vi "Template Build All.vi"(9 "Build Options":T1, 10 "Changes":string, 11 "Version Increment":T3) -> (1 "Build Error":bool, 2 "Status":string, 3 "Version":T2, 5 "Description":string)   [LabVIEW 2021]
uses:
  <vilib>/CIF Foundation/CIF LabVIEW Scripting/LV Scripting/Typedef/Version Increment.ctl
  <vilib>/CIF Foundation/CIF LabVIEW Scripting/LV Scripting/Typedef/Version.ctl
  Template Core Utilities/Typedef/Build Options.ctl
  Template Core Utilities/TemplateCoreUtilities.lvlib
  <vilib>/CIF Foundation/CIF LabVIEW Scripting/LV Scripting/LV Scripting Utilities.lvlib
panel:
  # "If built RT plugin has problems loading you may need to change the settings in the build spec for the RT plugin. These settings optimize memory footprint but can cause load issues in some cases."
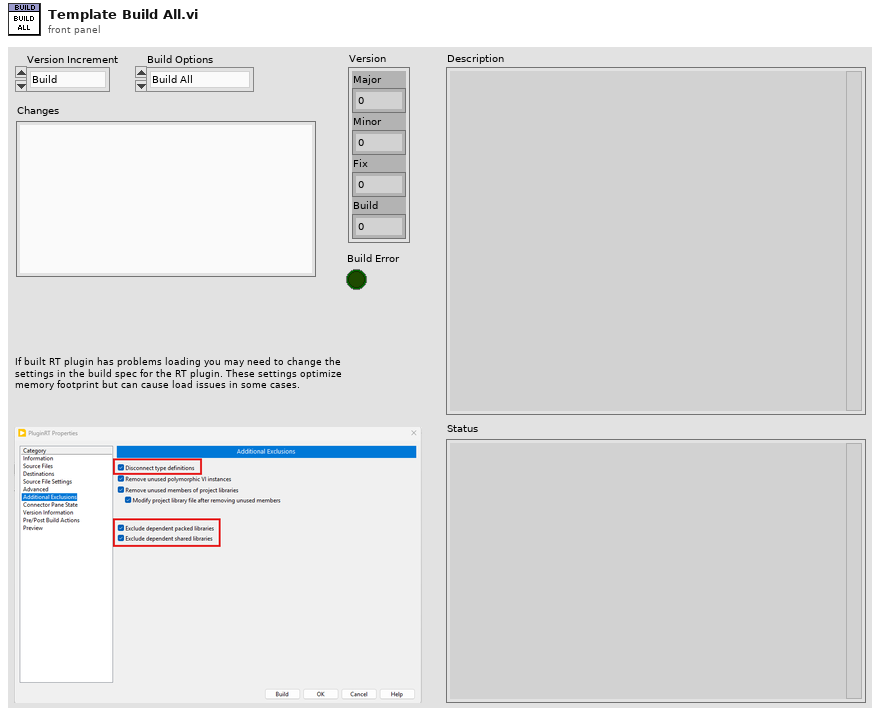
[diagram p1: front panel]
types:
  T1 = typedef "TemplateCoreUtilities.lvlib/Build Options.ctl" = enum16{"Build All", "Build RT Only", "Build Win Only", "Build UI Only"}
  T2 = typedef "Version.ctl" = cluster{"Major":u16, "Minor":u16, "Fix":u16, "Build":u16}
  T3 = typedef "LV Scripting Utilities.lvlib/Version Increment.ctl" = enum16{"Build", "Fix", "Minor", "Major"}
  T4 = typedef "TemplateCoreUtilities.lvlib/Calling VI References.ctl" = cluster{"Status":refnum<vi>, "Calling VI":refnum<vi>, "Description":refnum<vi>, "Version":refnum<vi>}
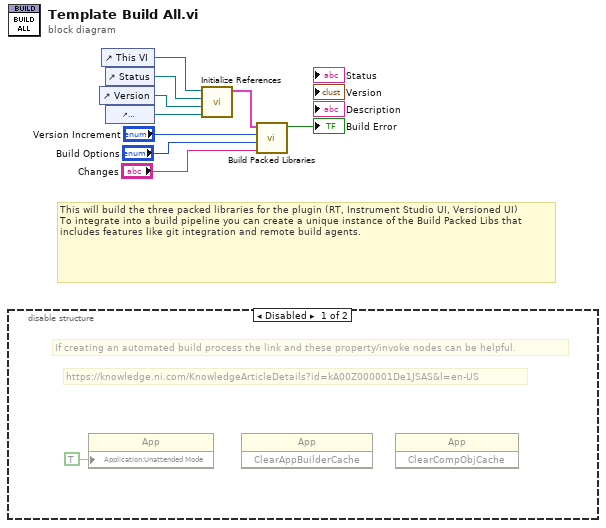
[diagram p0: block diagram]
diagram:
  # "This will build the three packed libraries for the plugin (RT, Instrument Studio UI, Versioned UI)\nTo integrate into a build pipeline you can create a unique instance of the Build Packed Libs that includes features like git integration and remote build agents."
  n1 = disable-structure shown="Disabled" {
    frame Disabled {
      # "If creating an automated build process the link and these property/invoke nodes can be helpful."
      # "https://knowledge.ni.com/KnowledgeArticleDetails?id=kA00Z000001De1JSAS&l=en-US"
      n2 = property class="App"("Application:Unattended Mode"=TRUE) -> ()  [unwired: 2 in, 2 out]
      n3 = invoke class="App" method="ClearAppBuilderCache"() -> ()  [unwired: 3 in, 3 out]
      n4 = invoke class="App" method="ClearCompObjCache"() -> ()  [unwired: 3 in, 3 out]
    }
    frame Enabled {
    }
  }
  n5 = control-ref of="Version"() -> (w7:refnum<vi>)
  n6 = control-ref of="This VI"() -> (w9:refnum<vi>)
  n7 = control-ref of="Status"() -> (w8:refnum<vi>)
  n8 = control-ref of="Description"() -> (w6:refnum<vi>)
  n9 = call "Initialize References.vi"("Description"=w6, "Version"=w7, "Status"=w8, "Calling VI"=w9) -> ("Calling VI References"=w5:T4)  [unwired: 7 in]
  n10 = call "Build Packed Libraries.vi"("Changes"="Changes", "Build Options"="Build Options", "Version Increment"="Version Increment", "Calling VI References"=w5) -> ("Build Error"=→"Build Error":bool)  [unwired: 7 in]
